vi "Cache.Set Transfers.vi"(10 "Transfers":refnum<class "Transfer.lvclass">[](array[class]), 11 "Cache in":refnum<class "Cache.lvclass">) -> (3 "Cache out":refnum<class "Cache.lvclass">)   [LabVIEW 2017, in "DSF.Engine.lvlib" / "Cache.lvclass"]
uses:
  Cache.lvclass
  Transfer/Transfer.lvclass
  Cache.lvclass/Cache.ctl
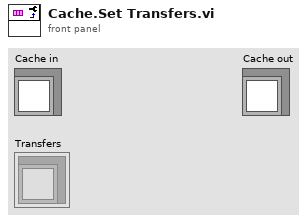
[diagram p1: front panel]
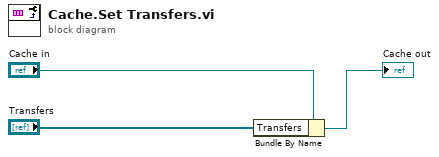
[diagram p0: block diagram]
diagram:
  n1 = Bundle By Name(cluster="Cache in", "Transfers"="Transfers") -> (→"Cache out":refnum<class "Cache.lvclass">)
